vi "GetReference2.vi"(0 "DeviceType":u32, 5 "DeviceInd":u32, 7 "CANInd":u32, 9 "RefType":T1 items=["REFTYPE_MODE"=0, "REFTYPE_FILTER"=1, "REFTYPE_ACR0"=2, "REFTYPE_AMR0"=6, "REFTYPE_kCANBAUD"=10, "REFTYPE_CANRX_EN"=13, "REFTYPE_UARTBAUD"=14, "REFTYPE_ALL"=15, "REFTYPE_BRS"=16], 11 "error in (no error)":errorcluster caption="错误输入（无错误）") -> (4 "Success":bool, 6 "Param":T2 {"ACR0" format="%x"}, 15 "error out":errorcluster caption="错误输出")   [LabVIEW 2011]
uses:
  VIs/Param.ctl
  VIs/ParamType.ctl
  data/ControlCAN.dll
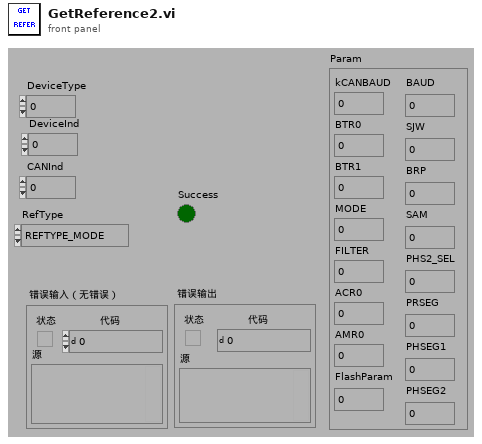
[diagram p1: front panel]
types:
  T1 = typedef "ParamType.ctl" = u32
  T2 = typedef "Param.ctl" = cluster{"kCANBAUD":u8, "BTR0":u8, "BTR1":u8, "MODE":u8, "FILTER":u8, "ACR0":u32, "AMR0":u32, "FlashParam":u32, "BAUD":u32, "SJW":u8, "BRP":u8, "SAM":u8, "PHS2_SEL":u8, "PRSEG":u8, "PHSEG1":u8, "PHSEG2":u8}
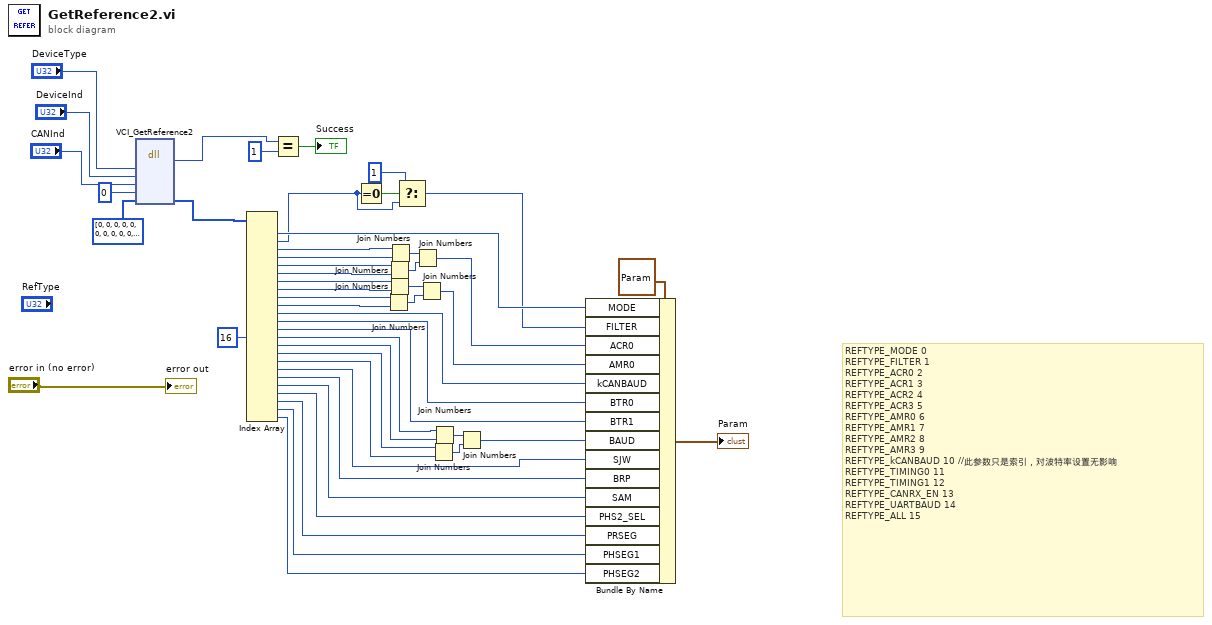
[diagram p0: block diagram]
diagram:
  # "REFTYPE_MODE 0\nREFTYPE_FILTER 1\nREFTYPE_ACR0 2\nREFTYPE_ACR1 3\nREFTYPE_ACR2 4\nREFTYPE_ACR3 5\nREFTYPE_AMR0 6\nREFTYPE_AMR1 7\nREFTYPE_AMR2 8\nREFTYPE_AMR3 9\nREFTYPE_kCANBAUD 10 //此参数只是索引，对波特率设置无影响\nREFTYPE_TIMING0 11\nREFTYPE_TIMING1 12\nREFTYPE_CANRX_EN 13\nREFTYPE_UARTBAUD 14\nREFTYPE_ALL 15"
  n1 = dll-call lib="PTH1Nabs D\t董海成\t上位机2.进行中USB-CAN TooldataControlCAN.dll" fn="VCI_GetReference2" label="VCI_GetReference"("DeviceType"="DeviceType", "DeviceInd"="DeviceInd", "CANInd"="CANInd", "RefType"=u32 0, "pData"=u8[] [0, 0, 0, 0, 0, 0, 0, 0, 0, 0, 0, 0, 0, 0, 0, 0, 0, 0, 0, 0, 0, 0, 0, 0, 0, 0, 0, 0, 0, 0, 0, 0]) -> ("返回类型"=w46:u32, "pData"=w41:u8[])  [unwired: 7 in, 2 out]
  n2 = Index Array(array=w41, index #14=16 ("索引")) -> (element #1=w36:u8, element #2=w3:u8, element #3=w33:u8, element #4=w32:u8, element #5=w31:u8, element #6=w30:u8, element #7=w26:u8, element #8=w25:u8, element #9=w24:u8, element #10=w23:u8, element #11=w21:u8, element #12=w20:u8, element #13=w19:u8, element #14=w16:u8, element #15=w15:u8, element #16=w14:u8, element #17=w13:u8, element #18=w11:u8, element #19=w10:u8, element #20=w9:u8, element #21=w8:u8, element #22=w7:u8, element #23=w6:u8, element #24=w5:u8)  [unwired: 23 in]
  n3 = Equal?(x=w46, y=u32 1) -> (x = y?=→"Success":bool)
  n4 = Equal To 0?(x=w3) -> (x = 0?=w4:bool)
  n5 = Join Numbers(hi=w24, lo=w23) -> ((hi.lo)=w27:u16)
  n6 = Join Numbers(hi=w31, lo=w30) -> ((hi.lo)=w35:u16)
  n7 = Join Numbers(hi=w26, lo=w25) -> ((hi.lo)=w28:u16)
  n8 = Join Numbers(hi=w33, lo=w32) -> ((hi.lo)=w34:u16)
  n9 = Select(t=u8 1, s=w4, f=w3) -> (s? t:f=w1:u8)
  n10 = Join Numbers(hi=w34, lo=w35) -> ((hi.lo)=w29:u32)
  n11 = Join Numbers(hi=w28, lo=w27) -> ((hi.lo)=w22:u32)
  n12 = Join Numbers(hi=w14, lo=w13) -> ((hi.lo)=w37:u16)
  n13 = Join Numbers(hi=w16, lo=w15) -> ((hi.lo)=w38:u16)
  n14 = Join Numbers(hi=w38, lo=w37) -> ((hi.lo)=w12:u32)
  n15 = Bundle By Name(cluster=T2 {"kCANBAUD"=0, "BTR0"=0, "BTR1"=0, "MODE"=0, "FILTER"=0, "ACR0"=0, "AMR0"=0, "FlashParam"=0, "BAUD"=0, "SJW"=0, "BRP"=0, "SAM"=0, "PHS2_SEL"=0, "PRSEG"=0, "PHSEG1"=0, "PHSEG2"=0} ("Param 2"), "MODE"=w36, "FILTER"=w1, "ACR0"=w29, "AMR0"=w22, "kCANBAUD"=w21, "BTR0"=w20, "BTR1"=w19, "BAUD"=w12, "SJW"=w11, "BRP"=w10, "SAM"=w9, "PHS2_SEL"=w8, "PRSEG"=w7, "PHSEG1"=w6, "PHSEG2"=w5) -> (→"Param":T2)
  "error out" <- "error in (no error)"
